vi "Teleop.vi"(10 "Match Info":T3={"Autonomous Elapsed Seconds"=0.0, "TeleOp Elapsed Seconds"=26.041, "Disabled Elapsed Seconds"=11.82, "Visited Autonomous"=FALSE, "Visited TeleOp"=TRUE, "Visited Disabled"=TRUE, "Autonomous Settings"={"Autonomous Style"=enum."Independent", "VI Refnum"=refnum}}, 11 "Call Context":T4=enum."Stop") -> ()   [LabVIEW 2020]
doc: "This VI is called for each TeleOp packet received from the DS where the robot is not disabled. It is often used to read from the joysticks and update I/O or to update setpoints for timed control loops. It should complete and return within 20 milliseconds or it may miss DS packets."
uses:
  <vilib>/Rock Robotics/WPI/DriverStation/WPI_DriverStationDerivedRobotMode.ctl
  <vilib>/Rock Robotics/WPI/DriverStation/WPI_DriverStationMatch Info.ctl
  <vilib>/Rock Robotics/WPI/ThirdParty/REV Robotics/REVLib/Typedef/Spark MAX Control Type.ctl
  <vilib>/Rock Robotics/WPI/ThirdParty/Sensors/navX/_TypeDefs/FRIC_navX_DeviceNumbersTypeDef.ctl
  <vilib>/Rock Robotics/WPI/ThirdParty/Phoenix-LabVIEW/CANCoder/Get/CTRE_Phoenix_CANcoder_GetSensorData.vi
  <vilib>/Rock Robotics/WPI/Utilities/WPI_GetSetVariantRefNum.vi
  <vilib>/addons/control/pid/pid.llb/PID (DBL).vi
  <vilib>/addons/control/pid/NI_PID_pid.lvlib
panel:
  out "Displacement":T1
  out "MPUTemp":dbl
  in  "dt (s)":dbl=-1.0 format="%.3f"
  out "Yaw":dbl=10.44
  in  "ScaleSpeed":dbl=0.5
  in  "PID gains 2":T2={"proportional gain (Kc)"=0.004667, "integral time (Ti, min)"=0.013, "derivative time (Td, min)"=0.0} {"derivative time (Td, min)" format="%.10f"; "integral time (Ti, min)" format="%.10f"; "proportional gain (Kc)" format="%.10f"}
  # "NOW WITH 200% MORE REV!!!!"
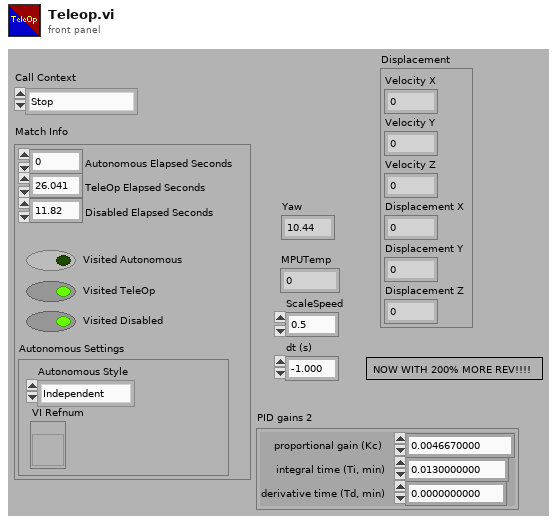
[diagram p1: front panel]
types:
  T1 = cluster{"Velocity X":dbl, "Velocity Y":dbl, "Velocity Z":dbl, "Displacement X":dbl, "Displacement Y":dbl, "Displacement Z":dbl}
  T2 = cluster{"proportional gain (Kc)":dbl, "integral time (Ti, min)":dbl, "derivative time (Td, min)":dbl}
  T3 = typedef "WPI_DriverStationMatch Info.ctl" = cluster{"Autonomous Elapsed Seconds":dbl, "TeleOp Elapsed Seconds":dbl, "Disabled Elapsed Seconds":dbl, "Visited Autonomous":bool, "Visited TeleOp":bool, "Visited Disabled":bool, "Autonomous Settings":cluster{"Autonomous Style":enum16{"Iterative", "Independent"}, "VI Refnum":refnum<vi>}}
  T4 = typedef "WPI_DriverStationDerivedRobotMode.ctl" = enum16{"Init", "Execute", "Stop"}
  T5 = typedef "FRIC_navX_DeviceNumbersTypeDef.ctl" = enum16{"Dev0", "Dev1", "Dev2", "Dev3"}
  T6 = typedef "Spark MAX Control Type.ctl" = enum16{"Percent VBus", "Voltage", "Velocity", "Position", "Smart Motion", "Current", "Smart Velocity"}
  T7 = typedef "WPI_JoystickDevRef.ctl" = cluster{"Device":T8}
  T8 = typedef "WPI_JoystickDeviceEnum.ctl" = enum16{"USB 0", "USB 1", "USB 2", "USB 3", "USB 4", "USB 5"}
  T9 = cluster{"Yaw":dbl, "Roll":dbl, "Pitch":dbl, "Heading":dbl, "Fused Heading":dbl}
  T10 = typedef "CTRE_Phoenix_CANcoder_DeviceRef.ctl" = cluster{"DeviceStatus":errorcluster, "Device Number":u8, "Handle":u64, "UsageFrame":u32, "Library Path":path}
  T11 = typedef "WPI_MotorControlDeviceRef.ctl" = cluster{"DeviceStatus":errorcluster, "Type":T12, "PWM":cluster{"PWM Channel":T13, "DeadBand":T14}, "CAN":cluster{"Device Number":u8, "SetOutput VI Ref":variant, "GetOutput VI Ref":variant, "Enable VI Ref":variant, "Disable VI Ref":variant, "Data":variant}, "Invert":bool, "DIO PWM":cluster{"PWM \"Enable\" Channel":T13, "DIOChannel":T15, "PWM Rate":dbl}}
  T12 = typedef "WPI_MotorControlType.ctl" = enum16{"PWM", "CAN", "DIO PWM"}
  T13 = typedef "FPGA_DIOPWMChannel.ctl" = enum8{"PWM 0", "PWM 1", "PWM 2", "PWM 3", "PWM 4", "PWM 5", "PWM 6", "PWM 7", "PWM 8", "PWM 9", "PWM MXP 0", "PWM MXP 1", "PWM MXP 2", "PWM MXP 3", "PWM MXP 4", "PWM MXP 5", "PWM MXP 6", "PWM MXP 7", "PWM MXP 8", "PWM MXP 9", "Invalid"}
  T14 = typedef "WPI_PWMDeadband.ctl" = cluster{"Name":string, "maxPositivePwm":i32, "minPositivePwm":i32, "centerPwm":i32, "maxNegativePwm":i32, "minNegativePwm":i32, "angularRange":u16}
  T15 = typedef "FPGA_DIOChannel.ctl" = enum8{"DIO 0", "DIO 1", "DIO 2", "DIO 3", "DIO 4", "DIO 5", "DIO 6", "DIO 7", "DIO 8", "DIO 9", "DIO MXP 0", "DIO MXP 1", "DIO MXP 2", "DIO MXP 3", "DIO MXP 4", "DIO MXP 5", "DIO MXP 6", "DIO MXP 7", "DIO MXP 8", "DIO MXP 9", "DIO MXP 10", "DIO MXP 11", "DIO MXP 12", "DIO MXP 13", "DIO MXP 14", "DIO MXP 15", "SPI Port CS1", "SPI Port CS2", "SPI Port CS3", "SPI Port MISO", "SPI Port MOSI", "Invalid"}
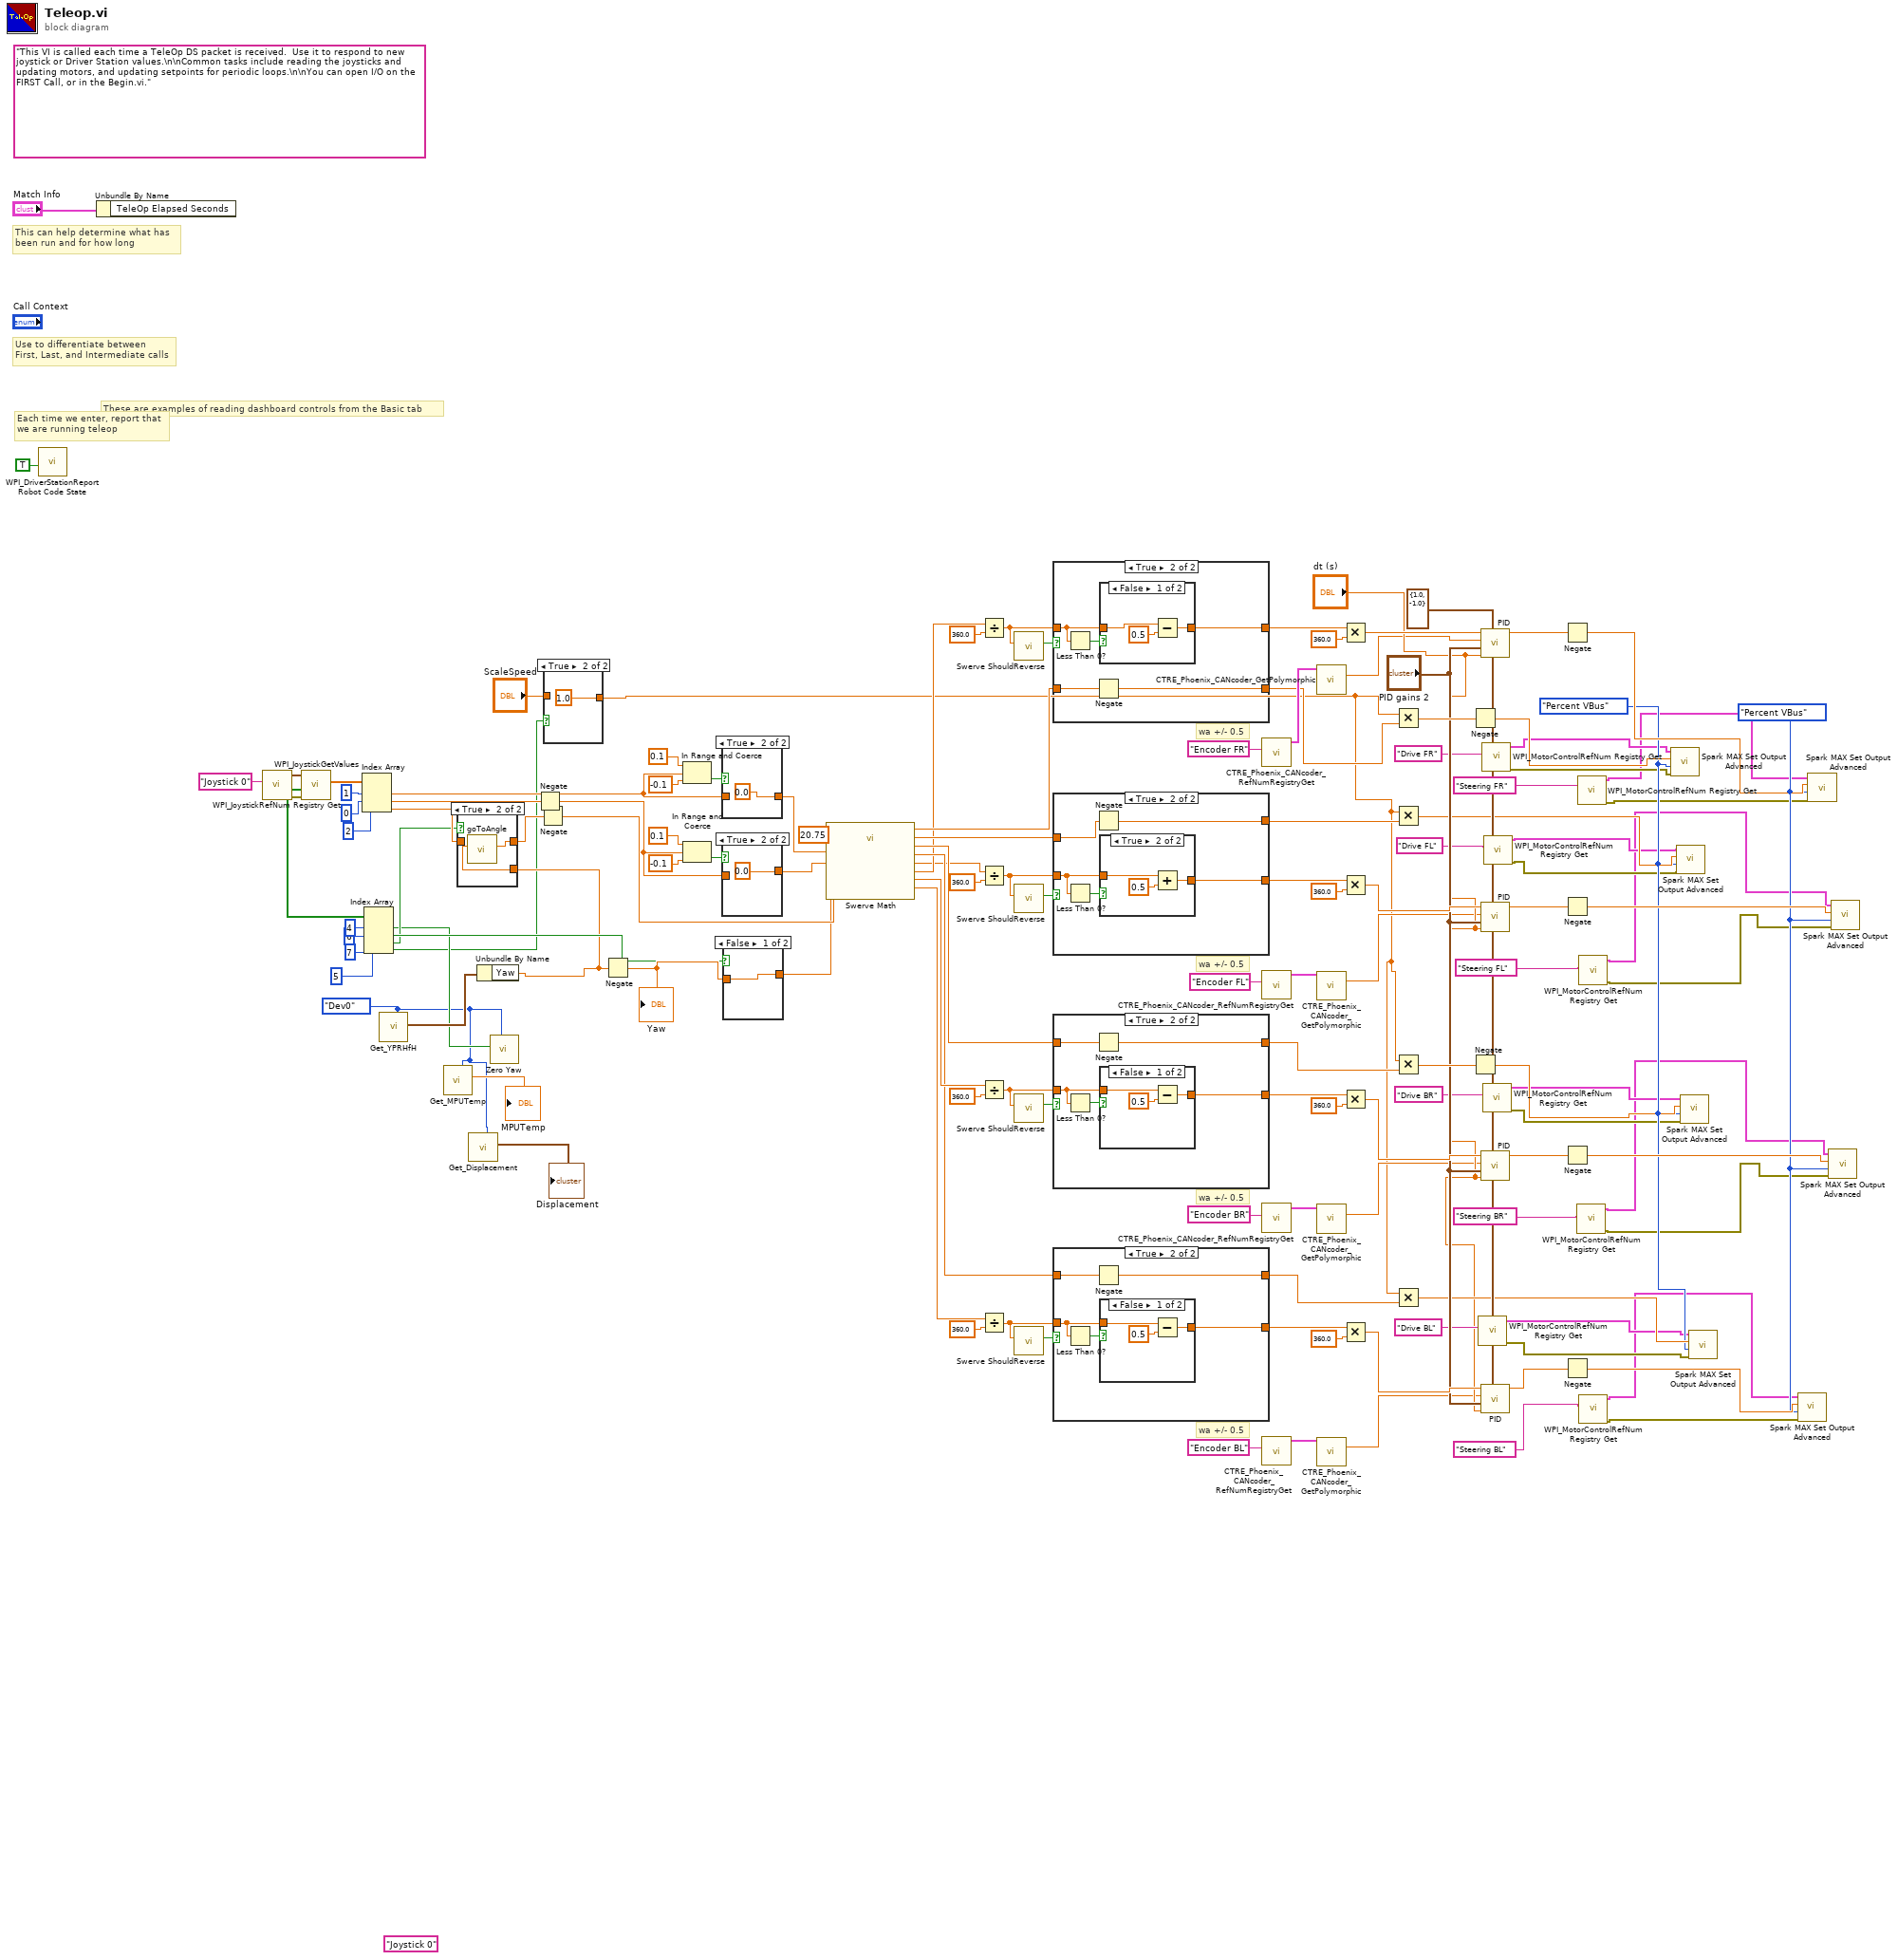
[diagram p0: block diagram]
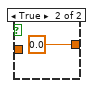
[diagram p4: hidden frame]
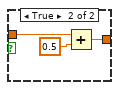
[diagram p6: hidden frame]
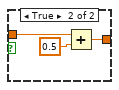
[diagram p8: hidden frame]
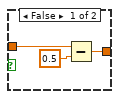
[diagram p10: hidden frame]
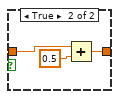
[diagram p12: hidden frame]
diagram:
  w6 = FRIC_navX_DeviceNumbersTypeDef."Dev0" ("Device Number")
  w56 = Spark_MAX_Control_Type."Percent VBus" ("Control Mode")
  w61 = Spark_MAX_Control_Type."Percent VBus" ("Control Mode")
  (unwired) "Joystick 0" ("refnum name")
  w66 = cluster{"output high":dbl, "output low":dbl} {"output high"=1.0, "output low"=-1.0} ("output range")
  w131 = 20.75 ("Trackwidth (W)")
  (unwired) "This VI is called each time a TeleOp DS packet is received.  Use it to respond to new joystick or Driver Station values.\n\nCommon tasks include reading the joysticks and updating motors, and updating setpoints for periodic loops.\n\nYou can open I/O on the FIRST Call, or in the Begin.vi."
  # "wa +/- 0.5"
  # "wa +/- 0.5"
  # "wa +/- 0.5"
  # "wa +/- 0.5"
  # "These are examples of reading dashboard controls from the Basic tab"
  # "Each time we enter, report that\nwe are running teleop"
  # "Use to differentiate between\nFirst, Last, and Intermediate calls"
  # "This can help determine what has\nbeen run and for how long"
  n1 = call <vilib>:"WPI_DriverStationReport Robot Code State.vi"("TeleOp"=TRUE ("Autonomous")) -> ()  [unwired: 10 in, 1 out]
  n2 = Unbundle By Name("Match Info") -> ()  [unwired: 1 out]
  n3 = call <vilib>:"WPI_JoystickRefNum Registry Get.vi"("refnum name"="Joystick 0") -> ("error out"=w127:errorcluster, "JoystickDevRef"=w126:T7)  [unwired: 9 in]
  n4 = call <vilib>:"WPI_JoystickGetValues.vi"("error in (no error)"=w127, "JoystickDevRef"=w126) -> ("Buttons"=w22:bool[], "Axes"=w124:dbl[])  [unwired: 5 in, 3 out]
  n5 = Index Array(array=w124, index #1=1 ("index"), index #2=0 ("index"), index #3=2 ("index")) -> (element #1=w115:dbl, element #2=w25:dbl, element #3=w11:dbl)
  n6 = Index Array(array=w22, index #1=4 ("index"), index #2=6 ("index"), index #3=7 ("index"), index #4=5 ("index")) -> (element #1=w8:bool, element #2=w16:bool, element #3=w10:bool, element #4=w1:bool)
  n7 = call <vilib>:"Get_YPRHfH.vi"("Device Number"=w6) -> ("YRPHfH"=w19:T9)  [unwired: 10 in]
  n8 = call <vilib>:"Get_MPUTemp.vi"("Device Number"=w6) -> ("MPUTemp"=→"MPUTemp":dbl)  [unwired: 10 in]
  n9 = call <vilib>:"Get_Displacement.vi"("Device Number"=w6) -> ("Displacement"=→"Displacement":T1)  [unwired: 10 in]
  n10 = Unbundle By Name(w19) -> ("Yaw"=w9:dbl)
  n11 = case shown="True" w10 {
    tunnel: [w134 w136] -> w12
    tunnel: w11 -> [w134 _]
    tunnel: w9 -> [_ w135]
    frame False {
    }
    frame True {
      n12 = call "goToAngle.vi"("gyro"=w135) -> ("x2"=w136:dbl)  [unwired: 10 in]
    }
  }
  n13 = call <vilib>:"Zero Yaw.vi"("Device Number"=w6, "Zero"=w8) -> ()  [unwired: 10 in]
  n14 = Negate(x=w25) -> (-x=w24:dbl)
  n15 = Negate(x=w12) -> (-x=w23:dbl)
  n16 = case shown="True" w1 {
    tunnel: [w137 1.0 ("upper limit")] -> w3
    tunnel: "ScaleSpeed" -> [w137 _]
    frame False {
    }
    frame True {
    }
  }
  n17 = Negate(x=w9) -> (-x=w17:dbl)
  "Yaw" <- w17
  n18 = In Range and Coerce(upper limit=0.1, x=w115, lower limit=-0.1) -> (In Range?=w119:bool)  [unwired: 1 out]
  n19 = In Range and Coerce(upper limit=0.1, x=w24, lower limit=-0.1) -> (In Range?=w118:bool)  [unwired: 1 out]
  n20 = case shown="True" w119 {
    tunnel: [w139 0.0 ("upper limit")] -> w113
    tunnel: w115 -> [w139 _]
    frame False {
    }
    frame True {
    }
  }
  n21 = case shown="True" w118 {
    tunnel: [w141 0.0 ("upper limit")] -> w114
    tunnel: w24 -> [w141 _]
    frame False {
    }
    frame True {
    }
  }
  n22 = case shown="False" w16 {
    tunnel: [w143 0.0 ("upper limit")] -> w18
    tunnel: w17 -> [w143 _]
    frame False {
    }
    frame True {
    }
  }
  n23 = call "Swerve Math.vi"("Trackwidth (W)"=w131, "Wheelbase (L)"=w131, "Y -FWD"=w113, "X1 STR"=w114, "X2 RCW"=w23, "Gyro Angle in degrees"=w18) -> ("wa3"=w70:dbl, "wa4"=w68:dbl, "ws1"=w73:dbl, "ws2"=w72:dbl, "ws3"=w71:dbl, "ws4"=w69:dbl, "wa2"=w15:dbl, "wa1"=w14:dbl)  [unwired: 2 in]
  n24 = Divide(x=w15, y=360.0) -> (x/y=w110:dbl)
  n25 = Divide(x=w14, y=360.0) -> (x/y=w99:dbl)
  n26 = Divide(x=w70, y=360.0) -> (x/y=w89:dbl)
  n27 = Divide(x=w68, y=360.0) -> (x/y=w78:dbl)
  n28 = call "Swerve ShouldReverse.vi"("wa in"=w110) -> ("shouldReverse out"=w111:bool)  [unwired: 10 in]
  n29 = call "Swerve ShouldReverse.vi"("wa in"=w99) -> ("shouldReverse out"=w100:bool)  [unwired: 10 in]
  n30 = call "Swerve ShouldReverse.vi"("wa in"=w89) -> ("shouldReverse out"=w90:bool)  [unwired: 10 in]
  n31 = call "Swerve ShouldReverse.vi"("wa in"=w78) -> ("shouldReverse out"=w79:bool)  [unwired: 10 in]
  n32 = case shown="True" w111 {
    tunnel: w73 -> [w146 w147]
    tunnel: w110 -> [w145 w150]
    tunnel: [w146 w148] -> w109
    tunnel: [w145 w149] -> w108
    frame False {
    }
    frame True {
      n33 = Less Than 0?(x=w150) -> (x < 0?=w151:bool)
      n34 = Negate(x=w147) -> (-x=w148:dbl)
      n35 = case shown="False" w151 {
        tunnel: w150 -> [w153 w156]
        tunnel: [w152 w155] -> w149
        frame False {
          n36 = Subtract(x=w153, y=0.5) -> (x-y=w152:dbl)
        }
        frame True {
          n37 = Add(x=w156, y=0.5) -> (x+y=w155:dbl)
        }
      }
    }
  }
  n38 = case shown="True" w100 {
    tunnel: w72 -> [w159 w160]
    tunnel: w99 -> [w158 w163]
    tunnel: [w159 w161] -> w98
    tunnel: [w158 w162] -> w97
    frame False {
    }
    frame True {
      n39 = Less Than 0?(x=w163) -> (x < 0?=w164:bool)
      n40 = Negate(x=w160) -> (-x=w161:dbl)
      n41 = case shown="True" w164 {
        tunnel: w163 -> [w166 w169]
        tunnel: [w165 w168] -> w162
        frame False {
          n42 = Subtract(x=w166, y=0.5) -> (x-y=w165:dbl)
        }
        frame True {
          n43 = Add(x=w169, y=0.5) -> (x+y=w168:dbl)
        }
      }
    }
  }
  n44 = case shown="True" w90 {
    tunnel: w71 -> [w172 w173]
    tunnel: w89 -> [w171 w176]
    tunnel: [w172 w174] -> w88
    tunnel: [w171 w175] -> w87
    frame False {
    }
    frame True {
      n45 = Less Than 0?(x=w176) -> (x < 0?=w177:bool)
      n46 = Negate(x=w173) -> (-x=w174:dbl)
      n47 = case shown="False" w177 {
        tunnel: w176 -> [w179 w182]
        tunnel: [w178 w181] -> w175
        frame False {
          n48 = Subtract(x=w179, y=0.5) -> (x-y=w178:dbl)
        }
        frame True {
          n49 = Add(x=w182, y=0.5) -> (x+y=w181:dbl)
        }
      }
    }
  }
  n50 = case shown="True" w79 {
    tunnel: w69 -> [w185 w186]
    tunnel: w78 -> [w184 w189]
    tunnel: [w185 w187] -> w77
    tunnel: [w184 w188] -> w76
    frame False {
    }
    frame True {
      n51 = Less Than 0?(x=w189) -> (x < 0?=w190:bool)
      n52 = Negate(x=w186) -> (-x=w187:dbl)
      n53 = case shown="False" w190 {
        tunnel: w189 -> [w192 w195]
        tunnel: [w191 w194] -> w188
        frame False {
          n54 = Subtract(x=w192, y=0.5) -> (x-y=w191:dbl)
        }
        frame True {
          n55 = Add(x=w195, y=0.5) -> (x+y=w194:dbl)
        }
      }
    }
  }
  n56 = call <vilib>:"CTRE_Phoenix_CANcoder_RefNumRegistryGet.vi"("refnum name"="Encoder FR") -> ("CTRE_CANcoder_DeviceRef"=w129:T10)  [unwired: 9 in, 1 out]
  n57 = call <vilib>:"CTRE_Phoenix_CANcoder_RefNumRegistryGet.vi"("refnum name"="Encoder FL") -> ("CTRE_CANcoder_DeviceRef"=w103:T10)  [unwired: 9 in, 1 out]
  n58 = call <vilib>:"CTRE_Phoenix_CANcoder_RefNumRegistryGet.vi"("refnum name"="Encoder BR") -> ("CTRE_CANcoder_DeviceRef"=w93:T10)  [unwired: 9 in, 1 out]
  n59 = call <vilib>:"CTRE_Phoenix_CANcoder_RefNumRegistryGet.vi"("refnum name"="Encoder BL") -> ("CTRE_CANcoder_DeviceRef"=w82:T10)  [unwired: 9 in, 1 out]
  n60 = call-poly <vilib>:"CTRE_Phoenix_CANcoder_GetPolymorphic.vi"("CTRE_CANcoder_DeviceRef"=w129) -> ("Position"=w27:dbl)  [unwired: 10 in, 4 out]
  n61 = call-poly <vilib>:"CTRE_Phoenix_CANcoder_GetPolymorphic.vi"("CTRE_CANcoder_DeviceRef"=w103) -> ("Position"=w28:dbl)  [unwired: 10 in, 4 out]
  n62 = call-poly <vilib>:"CTRE_Phoenix_CANcoder_GetPolymorphic.vi"("CTRE_CANcoder_DeviceRef"=w93) -> ("Position"=w29:dbl)  [unwired: 10 in, 4 out]
  n63 = call-poly <vilib>:"CTRE_Phoenix_CANcoder_GetPolymorphic.vi"("CTRE_CANcoder_DeviceRef"=w82) -> ("Position"=w26:dbl)  [unwired: 10 in, 4 out]
  n64 = Multiply(x=w108, y=360.0) -> (x*y=w107:dbl)
  n65 = Multiply(x=w97, y=360.0) -> (x*y=w96:dbl)
  n66 = Multiply(x=w87, y=360.0) -> (x*y=w86:dbl)
  n67 = Multiply(x=w76, y=360.0) -> (x*y=w75:dbl)
  n68 = Multiply(x=w3, y=w109) -> (x*y=w105:dbl)
  n69 = Multiply(x=w3, y=w98) -> (x*y=w59:dbl)
  n70 = Multiply(x=w3, y=w88) -> (x*y=w84:dbl)
  n71 = Multiply(x=w3, y=w77) -> (x*y=w57:dbl)
  n72 = Negate(x=w105) -> (-x=w60:dbl)
  n73 = Negate(x=w84) -> (-x=w58:dbl)
  n74 = call <vilib>:"WPI_MotorControlRefNum Registry Get.vi"("refnum name"="Drive BL") -> ("error out"=w36:errorcluster, "MotorControlDevRef"=w37:T11)  [unwired: 9 in]
  n75 = call-poly <vilib>:"PID.vi"("output range"=w66, "dt (s)"="dt (s)", "PID gains"="PID gains 2", "process variable"=w27, "setpoint"=w107) -> ("output"=w130:dbl)  [unwired: 5 in, 1 out]
  n76 = call-poly <vilib>:"PID.vi"("output range"=w66, "dt (s)"="dt (s)", "PID gains"="PID gains 2", "process variable"=w28, "setpoint"=w96) -> ("output"=w104:dbl)  [unwired: 5 in, 1 out]
  n77 = call-poly <vilib>:"PID.vi"("output range"=w66, "dt (s)"="dt (s)", "PID gains"="PID gains 2", "process variable"=w29, "setpoint"=w86) -> ("output"=w94:dbl)  [unwired: 5 in, 1 out]
  n78 = call-poly <vilib>:"PID.vi"("output range"=w66, "dt (s)"="dt (s)", "PID gains"="PID gains 2", "process variable"=w26, "setpoint"=w75) -> ("output"=w83:dbl)  [unwired: 5 in, 1 out]
  n79 = call <vilib>:"WPI_MotorControlRefNum Registry Get.vi"("refnum name"="Drive FR") -> ("error out"=w53:errorcluster, "MotorControlDevRef"=w54:T11)  [unwired: 9 in]
  n80 = call <vilib>:"WPI_MotorControlRefNum Registry Get.vi"("refnum name"="Drive BR") -> ("error out"=w41:errorcluster, "MotorControlDevRef"=w42:T11)  [unwired: 9 in]
  n81 = call <vilib>:"WPI_MotorControlRefNum Registry Get.vi"("refnum name"="Drive FL") -> ("error out"=w47:errorcluster, "MotorControlDevRef"=w48:T11)  [unwired: 9 in]
  n82 = Negate(x=w130) -> (-x=w65:dbl)
  n83 = Negate(x=w104) -> (-x=w64:dbl)
  n84 = Negate(x=w94) -> (-x=w63:dbl)
  n85 = Negate(x=w83) -> (-x=w62:dbl)
  n86 = call <vilib>:"WPI_MotorControlRefNum Registry Get.vi"("refnum name"="Steering BR") -> ("error out"=w39:errorcluster, "MotorControlDevRef"=w40:T11)  [unwired: 9 in]
  n87 = call <vilib>:"WPI_MotorControlRefNum Registry Get.vi"("refnum name"="Steering FR") -> ("error out"=w50:errorcluster, "MotorControlDevRef"=w51:T11)  [unwired: 9 in]
  n88 = call <vilib>:"WPI_MotorControlRefNum Registry Get.vi"("refnum name"="Steering FL") -> ("error out"=w44:errorcluster, "MotorControlDevRef"=w45:T11)  [unwired: 9 in]
  n89 = call <vilib>:"WPI_MotorControlRefNum Registry Get.vi"("refnum name"="Steering BL") -> ("error out"=w33:errorcluster, "MotorControlDevRef"=w34:T11)  [unwired: 9 in]
  n90 = call <vilib>:"Spark MAX Set Output Advanced.vi"("error in (no error)"=w53, "Control Mode"=w56, "Setpoint"=w60, "MotorControlDevRef"=w54) -> ()  [unwired: 6 in, 2 out]
  n91 = call <vilib>:"Spark MAX Set Output Advanced.vi"("error in (no error)"=w47, "Control Mode"=w56, "Setpoint"=w59, "MotorControlDevRef"=w48) -> ()  [unwired: 6 in, 2 out]
  n92 = call <vilib>:"Spark MAX Set Output Advanced.vi"("error in (no error)"=w41, "Control Mode"=w56, "Setpoint"=w58, "MotorControlDevRef"=w42) -> ()  [unwired: 6 in, 2 out]
  n93 = call <vilib>:"Spark MAX Set Output Advanced.vi"("error in (no error)"=w36, "Control Mode"=w56, "Setpoint"=w57, "MotorControlDevRef"=w37) -> ()  [unwired: 6 in, 2 out]
  n94 = call <vilib>:"Spark MAX Set Output Advanced.vi"("error in (no error)"=w33, "Control Mode"=w61, "Setpoint"=w62, "MotorControlDevRef"=w34) -> ()  [unwired: 6 in, 2 out]
  n95 = call <vilib>:"Spark MAX Set Output Advanced.vi"("error in (no error)"=w50, "Control Mode"=w61, "Setpoint"=w65, "MotorControlDevRef"=w51) -> ()  [unwired: 6 in, 2 out]
  n96 = call <vilib>:"Spark MAX Set Output Advanced.vi"("error in (no error)"=w39, "Control Mode"=w61, "Setpoint"=w63, "MotorControlDevRef"=w40) -> ()  [unwired: 6 in, 2 out]
  n97 = call <vilib>:"Spark MAX Set Output Advanced.vi"("error in (no error)"=w44, "Control Mode"=w61, "Setpoint"=w64, "MotorControlDevRef"=w45) -> ()  [unwired: 6 in, 2 out]
